vi "myFFT_ResultFilt.vi"(0 "可用PICO数":u16=2, 3 "响应选项":u8=2, 4 "写表结果输入":dbl[][](array[numeric]), 5 "注入选项":u8=2) -> (1 "写表结果输出":dbl[][](array[numeric]))   [LabVIEW 2024]
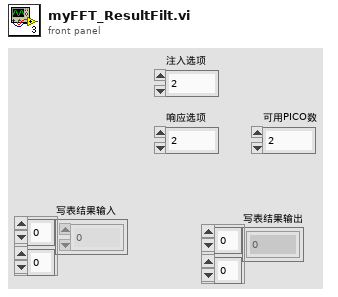
[diagram p1: front panel]
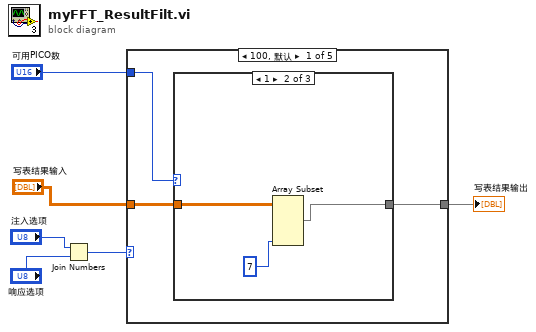
[diagram p0: block diagram]
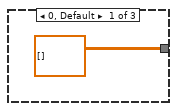
[diagram p2: hidden frame]
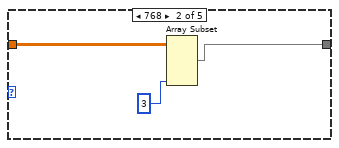
[diagram p4: hidden frame]
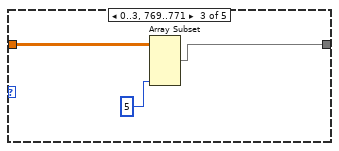
[diagram p5: hidden frame]
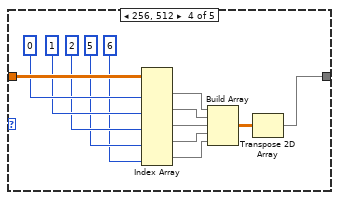
[diagram p6: hidden frame]
diagram:
  n1 = Join Numbers(hi="注入选项", lo="响应选项") -> ((hi.lo)=w4:u16)
  n2 = case shown="100, 默认" w4 {
    tunnel: "可用PICO数" -> [w9 _ _ _ _]
    tunnel: "写表结果输入" -> [w8 w17 w20 w33 w34]
    tunnel: [w7 w15 w19 w21 w34] -> w1
    frame 100, Default {
      n3 = case shown="1" w9 {
        tunnel: w8 -> [_ w13 w14]
        tunnel: [dbl[][] [] ("写表结果输入 2") w12 w14] -> w7
        frame 0, Default {
        }
        frame 1 {
          n4 = Array Subset(array=w13, length (col)=7 ("长度")) -> (w12:dbl[][])  [unwired: 3 in]
        }
        frame 2 {
        }
      }
    }
    frame 768 {
      n5 = Array Subset(array=w17, length (col)=3 ("长度")) -> (w15:dbl[][])  [unwired: 3 in]
    }
    frame 0..3, 769..771 {
      n6 = Array Subset(array=w20, length (col)=5 ("长度")) -> (w19:dbl[][])  [unwired: 3 in]
    }
    frame 256, 512 {
      n7 = Index Array(array=w33, index (col) #1=0 ("索引 (列)"), index (col) #2=1 ("索引 (列)"), index (col) #3=2 ("索引 (列)"), index (col) #4=5 ("索引 (列)"), index (col) #5=6 ("索引 (列)")) -> (element #1=w27:dbl[], element #2=w23:dbl[], element #3=w24:dbl[], element #4=w26:dbl[], element #5=w25:dbl[])  [unwired: 5 in]
      n8 = Build Array(w27, w23, w24, w26, w25) -> (w22:dbl[][])
      n9 = Transpose 2D Array(2D array=w22) -> (transposed array=w21:dbl[][])
    }
    frame 257..259, 513..515 {
    }
  }
  "写表结果输出" <- w1
